vi "Keithley_get_current.vi"(0 "VISA resource name":refnum<visa-resource-name>, 1 "Keithley Delay":u32, 11 "error in (no error)":errorcluster) -> (4 "VISA resource name out":refnum<visa-resource-name>, 6 "Keithley_Voltage":dbl, 10 "Keithley Read Status":bool, 15 "error out":errorcluster)   [LabVIEW 2018]
uses:
  <vilib>/Utility/error.llb/whitespace.ctl
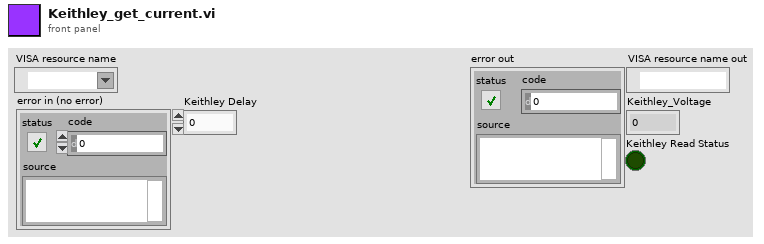
[diagram p1: front panel]
types:
  T1 = typedef "whitespace.ctl" = u16
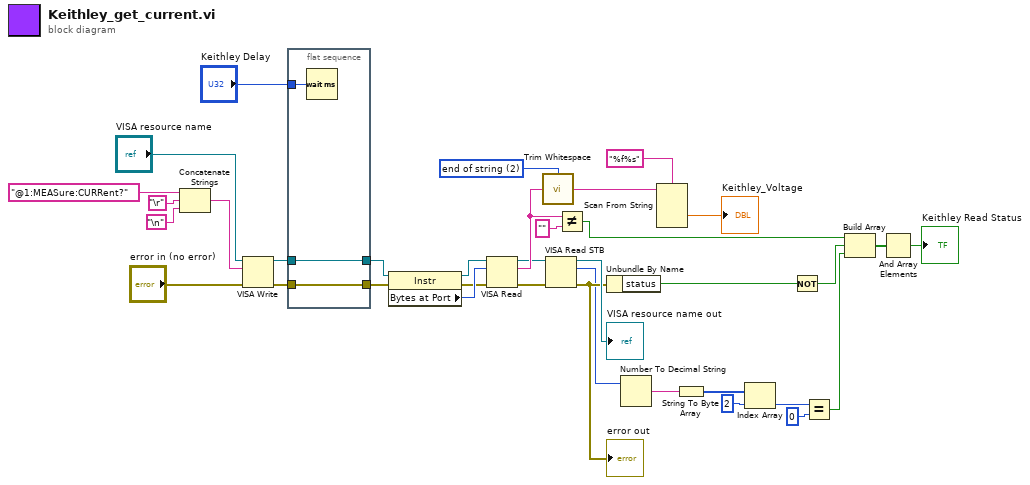
[diagram p0: block diagram]
diagram:
  w24 = T1 2 items=["both", "start of string", "end of string"] ("location (both)")
  n1 = Concatenate Strings("@1:MEASure:CURRent?" ("string"), "\r", "\n") -> (w33:string)
  n2 = VISA Write(VISA resource name="VISA resource name", write buffer=w33, error in (no error)="error in (no error)") -> (VISA resource name out=w32:refnum<visa-resource-name>, error out=w31:errorcluster)  [unwired: 1 out]
  n3 = flat-sequence {
    tunnel: w32 -> [w38]
    tunnel: w31 -> [w39]
    tunnel: [w39] -> w28
    tunnel: [w38] -> w29
    tunnel: "Keithley Delay" -> [w37]
    frame #0 {
      n4 = Wait (ms)(milliseconds to wait=w37) -> ()  [unwired: 1 out]
    }
  }
  n5 = property class="Instr"(reference=w29, error in=w28) -> (reference out=w27:refnum<visa-resource-name>, error out=w25:errorcluster, "Bytes at Port"=w26:u32)
  n6 = VISA Read(VISA resource name=w27, byte count=w26, error in (no error)=w25) -> (VISA resource name out=w15:refnum<visa-resource-name>, read buffer=w17:string, error out=w14:errorcluster)  [unwired: 1 out]
  n7 = call <vilib>:"Trim Whitespace.vi"("string"=w17, "location (both)"=w24) -> ("trimmed string"=w23:string)
  n8 = VISA Read STB(8:w14, 11:w15) -> (0:w12:errorcluster, 2:w11:u16, 3:→"VISA resource name out":refnum<visa-resource-name>)
  "error out" <- w12
  n9 = Not Equal?(x=w17, y="") -> (x != y?=w5:bool)
  n10 = Unbundle By Name(w12) -> ("status"=w20:bool)
  n11 = Number To Decimal String(number=w11) -> (decimal integer string=w10:string)  [unwired: 1 in]
  n12 = Scan From String(format string="%f%s", input string=w23) -> (output 1=→"Keithley_Voltage":dbl)  [unwired: 5 in, 3 out]
  n13 = String To Byte Array(string=w10) -> (unsigned byte array=w9:u8[])
  n14 = Index Array(array=w9, index=2) -> (element=w7:u8)
  n15 = Not(x=w20) -> (.not. x?=w4:bool)
  n16 = Equal?(x=w7, y=u8 0) -> (x = y?=w3:bool)
  n17 = Build Array(w5, w4, w3) -> (w2:bool[])
  n18 = And Array Elements(Boolean array=w2) -> (logical AND=→"Keithley Read Status":bool)
